vi "AutoStates.vi"(10 "AutoMode":T1, 11 "AutoState":T2) -> ()   [LabVIEW 2013]
uses:
  DoubleSolenoidAction.ctl
  SingleSolenoidAction.ctl
  AutoMode.ctl
  ServoAction.ctl
  AutoStates.ctl
panel:
  in  "ServoInitAngle":i32=140
  in  "error in (no error)":errorcluster
  out "error out":errorcluster
  in  "SwitchToLowGear?":bool
  # "SERVO"
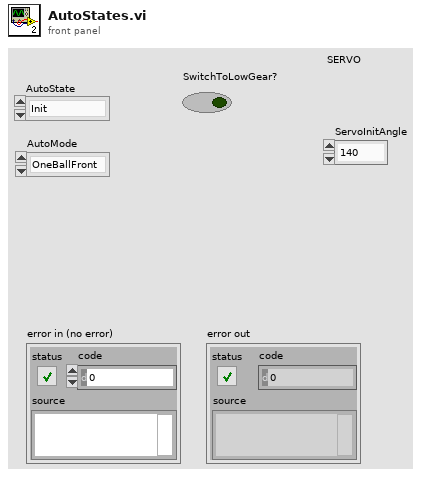
[diagram p1: front panel]
types:
  T1 = typedef "AutoMode.ctl" = enum16{"OneBallFront", "OneBallCollector", "TwoBallNormal", "TwoBallHot"}
  T2 = typedef "AutoStates.ctl" = enum16{"Init", "LowerArm", "CheckGoal", "DriveBack", "Collect", "StopCollect", "LiftArm", "RaiseServo", "Drive", "ShouldWait", "Wait", "ShootCollectorUp", "RaiseArm", "ShootCollectorDown", "Rotate1", "Rotate2", "Stop"}
  T3 = typedef "ServoAction.ctl" = enum16{"Init", "SetAngle", "GetAngle", "Lower", "Raise", "Disable"}
  T4 = typedef "DoubleSolenoidAction.ctl" = enum16{"Init", "Middle", "In", "Out"}
  T5 = typedef "SingleSolenoidAction.ctl" = enum16{"Init", "SetState", "Disable"}
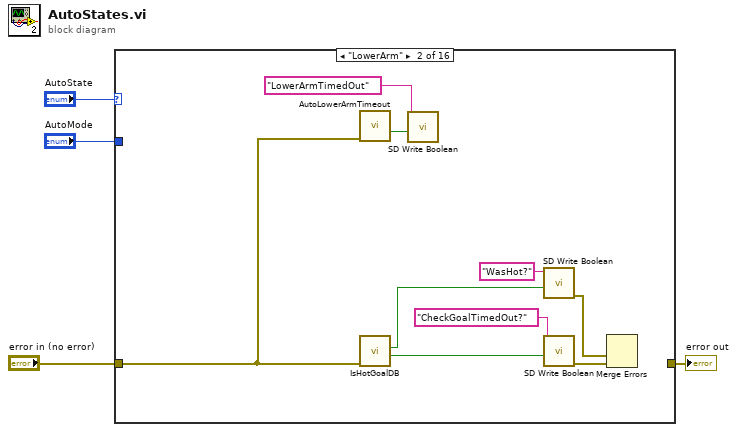
[diagram p0: block diagram]
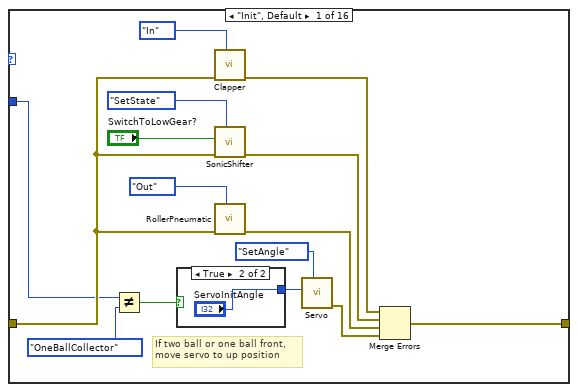
[diagram p2: hidden frame]
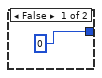
[diagram p3: hidden frame]
diagram:
  n1 = case shown="\"LowerArm\"" "AutoState" {
    tunnel: "AutoMode" -> [w14 _ _ _ _ _ _ _ _ _ _ _ _ _ _ _]
    tunnel: [w16 _ _ _ _ _ _ _ _ _ _ _ _ _ _ _] -> w1
    tunnel: "error in (no error)" -> [w15 w28 _ _ _ _ _ _ _ _ _ _ _ _ _ _]
    frame "Init", Default {
      # "If two ball or one ball front, \nmove servo to up position"
      n2 = Not Equal?(x=w14, y=AutoMode."OneBallCollector") -> (x != y?=w6:bool)
      n3 = case shown="True" w6 {
        tunnel: [0 "ServoInitAngle"] -> w12
        frame False {
        }
        frame True {
        }
      }
      n4 = call "Clapper.vi"("State"=DoubleSolenoidAction."In", "Error in"=w15) -> ("Error out"=w7:errorcluster)  [unwired: 9 in]
      n5 = call "SonicShifter.vi"("Action"=SingleSolenoidAction."SetState", "error in (no error)"=w15, "Actuate?"="SwitchToLowGear?") -> ("error out"=w8:errorcluster)  [unwired: 8 in]
      n6 = call "RollerPneumatic.vi"("State"=DoubleSolenoidAction."Out", "Error in"=w15) -> ("Error out"=w9:errorcluster)  [unwired: 9 in]
      n7 = call "Servo.vi"("Action"=ServoAction."SetAngle", "Angle (deg)"=w12) -> ("error out"=w10:errorcluster)  [unwired: 8 in, 1 out]
      n8 = Merge Errors(w7, w8, w9, w10) -> (w16:errorcluster)
    }
    frame "LowerArm" {
      n9 = call "AutoLowerArmTimeout.vi"("error in (no error)"=w28) -> ("TimedOut?"=w29:bool)  [unwired: 9 in, 1 out]
      n10 = call "IsHotGoalDB.vi"("error in"=w28) -> ("TimedOut?"=w26:bool, "Hot?"=w24:bool)  [unwired: 8 in, 1 out]
      n11 = call <vilib>:"SD Write Boolean.vi"("Boolean"=w29, "Name"="LowerArmTimedOut") -> ()  [unwired: 8 in, 2 out]
      n12 = call <vilib>:"SD Write Boolean.vi"("Boolean"=w24, "Name"="WasHot?") -> ("error out"=w22:errorcluster)  [unwired: 8 in, 1 out]
      n13 = call <vilib>:"SD Write Boolean.vi"("Boolean"=w26, "Name"="CheckGoalTimedOut?") -> ("error out"=w23:errorcluster)  [unwired: 8 in, 1 out]
      n14 = Merge Errors(w22, w23) -> ()  [unwired: 2 in, 1 out]
    }
    frame "DriveBack" {
    }
    frame "Collect" {
    }
    frame "StopCollect" {
    }
    frame "LiftArm" {
    }
    frame "RaiseServo" {
    }
    frame "Drive" {
    }
    frame "ShouldWait" {
    }
    frame "Wait" {
    }
    frame "ShootCollectorUp" {
    }
    frame "RaiseArm" {
    }
    frame "ShootCollectorDown" {
    }
    frame "Rotate1" {
    }
    frame "Rotate2" {
    }
    frame "Stop" {
    }
  }
  "error out" <- w1
